vi "NiFPGA Close.vi"(7 "Attribute":T1, 8 "error in (no error)":errorcluster, 11 "Session":u32) -> (0 "error out":errorcluster, 3 "Session Out":u32)   [LabVIEW 2010, in "FPGA Interface Wrapper.lvlib"]
doc: "Closes the session to the FPGA. The FPGA resets unless either another session is still open or you use the NiFpga_CloseAttribute_NoResetIfLastSession attribute."
uses:
  <userlib>/_FPGA Interface Advanced Tools/FPGA Interface Wrapper/FPGA Interface Wrapper.lvlib
  <userlib>/_FPGA Interface Advanced Tools/FPGA Interface Wrapper/TypeDefs/Close Attribute.ctl
  NiFpga.dll
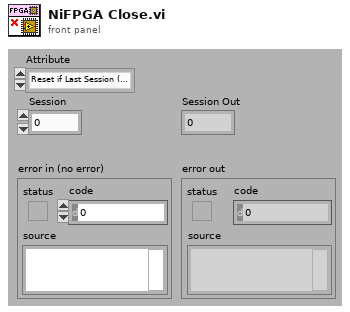
[diagram p1: front panel]
types:
  T1 = typedef "FPGA Interface Wrapper.lvlib/Close Attribute.ctl" = enum32{"Reset if Last Session (Default)", "No Reset"}
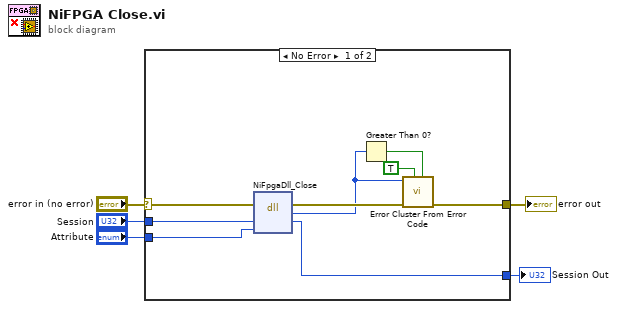
[diagram p0: block diagram]
diagram:
  n1 = case shown="No Error" "error in (no error)" {
    selector: "error in (no error)" -> [w14 w15]
    tunnel: [w7 w15] -> w4
    tunnel: "Session" -> [w13 w16]
    tunnel: [w12 w16] -> w2
    tunnel: "Attribute" -> [w11 _]
    frame No Error {
      n2 = dll-call lib="NiFpga.dll" fn="NiFpgaDll_Close"(error in=w14, "Session"=w13, "Attribute"=w11) -> (error out=w8:errorcluster, "Status"=w6:i32, "Session"=w12:u32)  [unwired: 3 in, 1 out]
      n3 = Greater Than 0?(x=w6) -> (x > 0?=w9:bool)
      n4 = call <vilib>:"Error Cluster From Error Code.vi"("is warning? (False)"=w9, "show call chain? (False)"=TRUE, "error in (no error)"=w8, "error code (0)"=w6) -> ("error out"=w7:errorcluster)  [unwired: 5 in]
    }
    frame Error {
    }
  }
  "error out" <- w4
  "Session Out" <- w2
